vi "GetStringData.vi"(8 "error in (no error)":errorcluster caption="Fehler (Eingang, kein Fehler)", 10 "Name":string, 11 "DictionaryString Eingang":refnum<class "DictionaryString.lvclass"> caption="DNL_LabVIEW Object in") -> (0 "error out":errorcluster caption="Fehler (Ausgang)", 2 "Value":string, 3 "DictionaryString Ausgang":refnum<class "DictionaryString.lvclass"> caption="DNL_LabVIEW Object out")   [LabVIEW 2013, in "LvDictionary.lvlib" / "DictionaryString.lvclass"]
uses:
  DictionaryString.lvclass
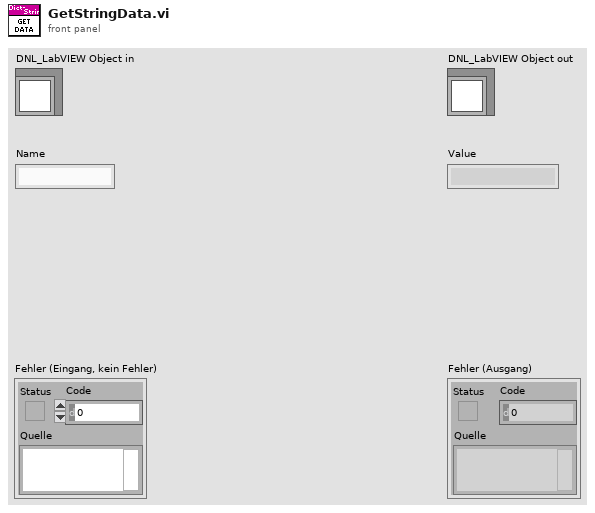
[diagram p1: front panel]
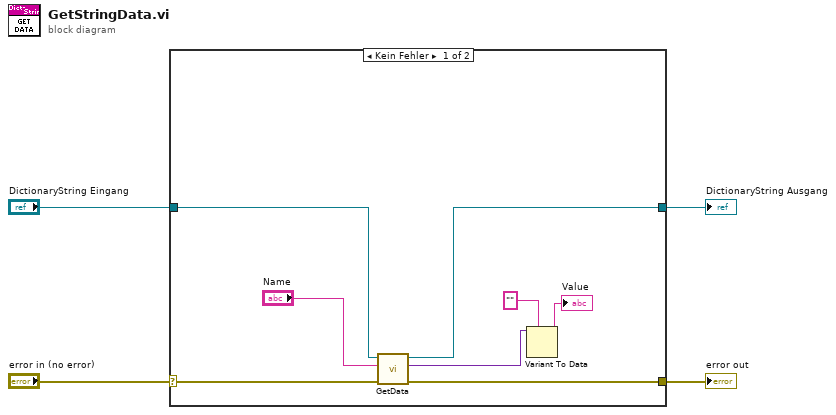
[diagram p0: block diagram]
diagram:
  n1 = case shown="Kein Fehler" "error in (no error)" {
    selector: "error in (no error)" -> [w8 w14]
    tunnel: "DictionaryString Eingang" -> [w11 w13]
    tunnel: [w10 w13] -> w2
    tunnel: [w9 w14] -> w1
    frame No Error {
      n2 = call-dynamic "GetData.vi"("error in (no error)"=w8, "Name"="Name", "Dictionary Eingang"=w11) -> ("error out"=w9:errorcluster, "Wert"=w6:variant, "Dictionary Ausgang"=w10:refnum<class "DictionaryString.lvclass">)  [unwired: 6 in]
      n3 = Variant To Data(type="" ("Typ"), Variant=w6) -> (data=→"Value":string)  [unwired: 1 in, 1 out]
    }
    frame Error {
    }
  }
  "error out" <- w1
  "DictionaryString Ausgang" <- w2
